vi "Dialogue - One Button.vi"(11 "Message":string) -> ()   [LabVIEW 2015, in "Utility.lvlib"]
uses:
  Utility.lvlib
  UI/System Button (without mouse hover).ctl
panel:
  in  "True Button":T1
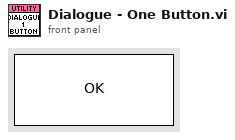
[diagram p1: front panel]
types:
  T1 = typedef "Utility.lvlib/System Button (without mouse hover).ctl" = bool
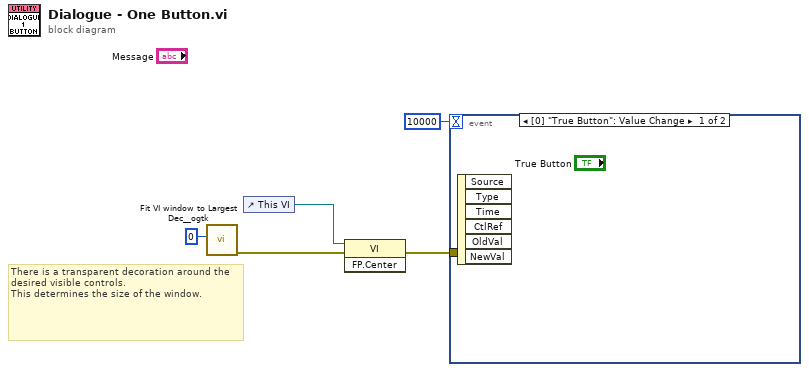
[diagram p0: block diagram]
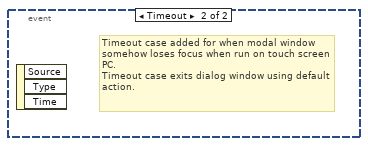
[diagram p2: hidden frame]
diagram:
  # "There is a transparent decoration around the desired visible controls.\nThis determines the size of the window."
  n1 = call <userlib>:"Fit VI window to Largest Dec__ogtk.vi"("border spacing (2 px)"=0) -> ("error out"=w3:errorcluster)  [unwired: 2 in, 4 out]
  n2 = control-ref of="This VI"() -> (w4:refnum<vi>)
  n3 = invoke class="VI" method="FP.Center"(reference=w4, error in=w3) -> (error out=w2:errorcluster)  [unwired: 1 in, 2 out]
  n4 = event shown="[0] \"True Button\": Value Change" {
    selector: _ -> [_ _]
    dyn-events: _ -> [_ _]
    timeout: 10000 -> [_ _]
    tunnel: w2 -> [_ _]
    event Value Change {
      n5 = event-data() -> ()  [unwired: 1 in, 6 out]
    }
    event Timeout {
      # "Timeout case added for when modal window somehow loses focus when run on touch screen PC.\nTimeout case exits dialog window using default action."
      n6 = event-data() -> ()  [unwired: 1 in, 3 out]
    }
  }
